vi "VI Stoermeldung Konfig.vi"() -> ()   [LabVIEW 2020, in "Stoerungen.lvlib"]
uses:
  Stoerungen/Stoerungen.lvlib
  Stoerungen/Stoermeldung Konfig Anzeige.ctl
  Stoerungen/Stoermeldung Konfig.ctl
  Visualisierungs Elemente/Zahlen-Ausgabefeld.ctl
  Visualisierungs Elemente/Zahlen-Eingabefeld.ctl
  Visualisierungs Elemente/String - Ausgabefeld.ctl
  Visualisierungs Elemente/Button.ctl
  Sprachverwaltung/FGV Aktion Tabelle zerlegen.ctl
  Passwortverwaltung/FGV Passwort Aktion.ctl
  Stoerungen/FGV Stoerungsdatei Aktionen.ctl
  Stoerungen/FGV Stoerung aufnehmen Aktion.ctl
  Passwortverwaltung/Passwort.lvlib
  Allgemein/allgemeine Sub-VIs.lvlib
  Sprachverwaltung/Sprachverwaltung.lvlib
panel:
  in  "Speichern":T1
  in  "Konfig":T2 {"Ansprech" format="%#_5g"; "Nummer" format="%#_5g"}
  # "Störmeldungs-Konfiguration"
  # "Störungs-\nNummer"
  # "Ansprech-\nverzögerung"
  # "Quittieren"
  # "Abschalten"
  # "Meldung"
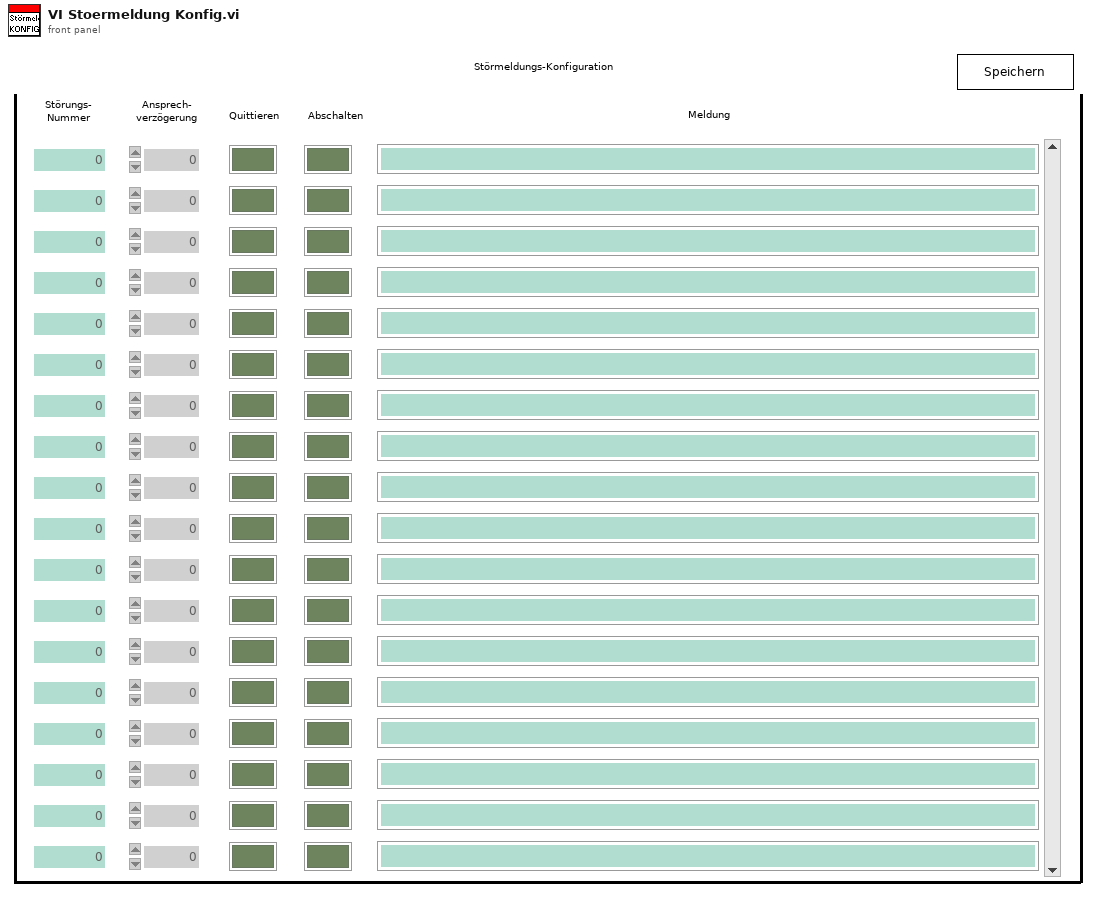
[diagram p1: front panel]
types:
  T1 = typedef "Button.ctl" = bool
  T2 = typedef "Stoerungen.lvlib/Stoermeldung Konfig Anzeige.ctl" = T3[]
  T3 = typedef "Stoerungen.lvlib/Stoermeldung Konfig.ctl" = cluster{"Quitt":bool, "Stopp":bool, "Nummer":T4, "Ansprech":T5, "Meldung":T6}
  T4 = typedef "Zahlen-Ausgabefeld.ctl" = sgl
  T5 = typedef "Zahlen-Eingabefeld.ctl" = sgl
  T6 = typedef "String - Ausgabefeld.ctl" = string
  T7 = typedef "Sprachverwaltung.lvlib/FGV Aktion Tabelle zerlegen.ctl" = enum16{"laden", "vereinzeln", "speichern"}
  T8 = typedef "Passwort.lvlib/FGV Passwort Aktion.ctl" = enum16{"prüfen", "setzen", "Initialisieren", "PW speichern", "lesen", "PW Änderung"}
  T9 = enum16{"open", "replace", "create", "open or create", "replace or create", "replace or create with confirmation"}
  T10 = typedef "Stoerungen.lvlib/FGV Stoerungsdatei Aktionen.ctl" = enum16{"lesen", "laden", "Neue Werte"}
  T11 = typedef "Stoerungen.lvlib/FGV Stoerung aufnehmen Aktion.ctl" = enum16{"Initialisieren", "Schreiben", "Lesen", "Quittieren", "quit. löschen"}
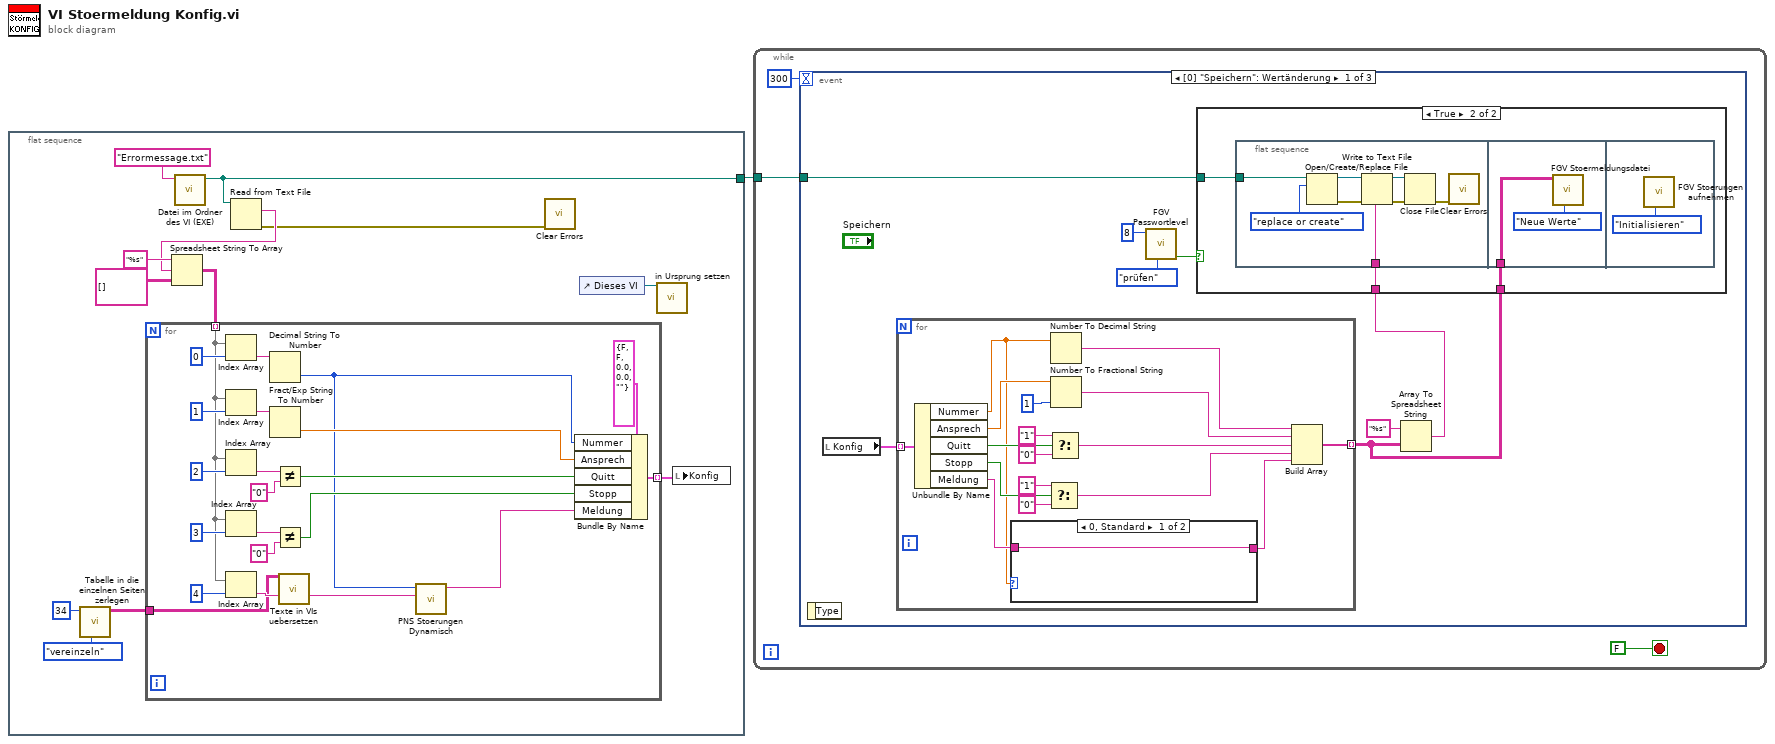
[diagram p0: block diagram]
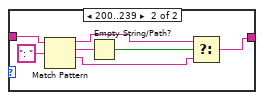
[diagram p3: hidden frame]
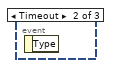
[diagram p4: hidden frame]
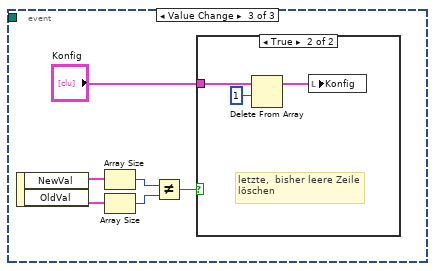
[diagram p5: hidden frame]
diagram:
  n1 = flat-sequence {
    tunnel: [w9] -> w1
    frame #0 {
      n2 = call "Tabelle in die einzelnen Seiten zerlegen.vi"("Aktion"=FGV_Aktion_Tabelle_zerlegen."vereinzeln", "Index (Seite)"=34) -> ("Sprachliste"=w3:string[][])  [unwired: 7 in, 2 out]
      n3 = call "Datei im Ordner des VI (EXE).vi"("Dateiname"="Errormessage.txt") -> ("Dateipfad im Ordner des Haupt-VIs"=w9:path)  [unwired: 8 in, 2 out]
      n4 = Read from Text File(file (use dialog)=w9) -> (text=w7:string, error out=w6:errorcluster)  [unwired: 1 in, 4 out]
      n5 = Spreadsheet String To Array(format string="%s" ("Format-String"), spreadsheet string=w7, array type (2D Dbl)=string[][] []) -> (array=w10:string[][])  [unwired: 1 out]
      n6 = for {
        tunnel: w10 -> [w27] mode=indexing
        tunnel: [w19] -> w8 mode=indexing
        tunnel: w3 -> [w17]
        n7 = Index Array(array=w27, index=0 ("Index")) -> (element=w24:string)
        n8 = Index Array(array=w27, index=1 ("Index")) -> (element=w31:string)
        n9 = Index Array(array=w27, index=2 ("Index")) -> (element=w34:string)
        n10 = Index Array(array=w27, index=3 ("Index")) -> (element=w30:string)
        n11 = Index Array(array=w27, index=4 ("Index")) -> (element=w18:string)
        n12 = Decimal String To Number(string=w24) -> (number=w15:i32)  [unwired: 3 out]
        n13 = Fract/Exp String To Number(string=w31) -> (number=w22:dbl)  [unwired: 4 out]
        n14 = Not Equal?(x=w34, y="0") -> (x != y?=w21:bool)
        n15 = Not Equal?(x=w30, y="0") -> (x != y?=w20:bool)
        n16 = call "Texte in VIs uebersetzen.vi"("Sprachliste"=w17, "String zum Übersetzen"=w18) -> ("String zum Übersetzen"=w16:string)  [unwired: 9 in, 4 out]
        n17 = call "PNS Stoerungen Dynamisch.vi"("Störmeldetexte"=w16, "Nummer"=w15) -> ("String"=w14:string)  [unwired: 9 in]
        n18 = Bundle By Name(cluster=T3 {"Quitt"=FALSE, "Stopp"=FALSE, "Nummer"=0.0, "Ansprech"=0.0, "Meldung"=""} ("Störmeldung Konfig"), "Nummer"=w15, "Ansprech"=w22, "Quitt"=w21, "Stopp"=w20, "Meldung"=w14) -> (w19:T3)
      }
      n19 = call <vilib>:"Clear Errors.vi"("error in (no error)"=w6) -> ()  [unwired: 5 in, 2 out]
      n20 = control-ref of="Dieses VI"() -> (w5:refnum<vi>)
      n21 = call "in Ursprung setzen.vi"("VI Referenz"=w5) -> ()  [unwired: 10 in, 1 out]
      n22 = local write "Konfig"(w8) -> ()
    }
  }
  n23 = while {
    tunnel: w1 -> [w38]
    stop <- FALSE stop-if-true
    n24 = event shown="[0] \"Speichern\": Wertänderung" {
      selector: _ -> [_ _ _]
      dyn-events: _ -> [_ _ _]
      timeout: 300 -> [_ _ _]
      tunnel: w38 -> [w46 _ _]
      event Value Change {
        n25 = event-data() -> ()  [unwired: 2 out]
        n26 = local read "Konfig"() -> (w43:T2)
        n27 = for {
          tunnel: [w77] -> w39 mode=indexing
          tunnel: w43 -> [w76] mode=indexing
          n28 = Unbundle By Name(w76) -> ("Nummer"=w62:T4, "Ansprech"=w73:T5, "Quitt"=w75:bool, "Stopp"=w74:bool, "Meldung"=w63:T6)
          n29 = case shown="0, Standard" w62 {
            tunnel: w63 -> [w78 w84]
            tunnel: [w78 w80] -> w61
            frame 0, Default {
            }
            frame 200..239 {
              n30 = Match Pattern(string=w84, regular expression=": " ("Regulärer Ausdruck")) -> (before substring=w82:T6, match substring=w81:T6, after substring=w79:T6)  [unwired: 1 in, 1 out]
              n31 = Empty String/Path?(string/path=w81) -> (empty?=w83:bool)
              n32 = Select(t=w82, s=w83, f=w79) -> (s? t:f=w80:T6)
            }
          }
          n33 = Select(t="1", s=w74, f="0") -> (s? t:f=w64:string)
          n34 = Select(t="1", s=w75, f="0") -> (s? t:f=w65:string)
          n35 = Number To Decimal String(number=w62) -> (decimal integer string=w72:string)  [unwired: 1 out]
          n36 = Number To Fractional String(number=w73, precision (6)=i16 1 ("Genauigkeit (6)")) -> (F-format string=w67:string)  [unwired: 2 out]
          n37 = Build Array(w72, w67, w65, w64, w61) -> (w77:T6[])
        }
        n38 = call "FGV Passwortlevel.vi"("FGV Passwort Aktion"=FGV_Passwort_Aktion."prüfen", "geforderter Level"=i16 8) -> ("Freigabe"=w41:bool)  [unwired: 2 in, 7 out]
        n39 = Array To Spreadsheet String(array=w39, 3:"%s" ("Format-String")) -> (spreadsheet string=w44:string)  [unwired: 1 out]
        n40 = case shown="True" w41 {
          tunnel: w46 -> [_ w49]
          tunnel: w44 -> [_ w48]
          tunnel: w39 -> [_ w47]
          frame False {
          }
          frame True {
            n41 = flat-sequence {
              tunnel: w49 -> [w57]
              tunnel: w48 -> [w56]
              tunnel: w47 -> [w58]
              frame #0 {
                n42 = Open/Create/Replace File(file path (use dialog)=w57, operation (0:open)=T9."replace or create" ("Operation (0:Öffnen)")) -> (refnum out=w53:refnum<file>, error out=w52:errorcluster)  [unwired: 1 in, 4 out]
                n43 = Write to Text File(file (use dialog)=w53, text=w56, error in=w52) -> (refnum out=w55:refnum<file>, error out=w51:errorcluster)  [unwired: 2 out]
                n44 = Close File(refnum=w55, error in=w51) -> (error out=w50:errorcluster)  [unwired: 1 out]
                n45 = call <vilib>:"Clear Errors.vi"("error in (no error)"=w50) -> ()  [unwired: 5 in, 2 out]
              }
              frame #1 {
                n46 = call "FGV Stoermeldungsdatei.vi"("Aktionen"=FGV_Stoerungsdatei_Aktionen."Neue Werte", "Neue Tabelle"=w58) -> ()  [unwired: 1 in, 9 out]
              }
              frame #2 {
                n47 = call "FGV Stoerungen aufnehmen.vi"("FGV Störung aufnehmen Aktion"=FGV_Stoerung_aufnehmen_Aktion."Initialisieren") -> ()  [unwired: 7 in, 4 out]
              }
            }
          }
        }
      }
      event Timeout {
        n48 = event-data() -> ()  [unwired: 2 out]
      }
      event Value Change {
        n49 = event-data() -> ("NewVal"=w91:T2, "OldVal"=w90:T2)  [unwired: 1 out]
        n50 = Array Size(array=w91) -> (size(s)=w89:i32)
        n51 = Array Size(array=w90) -> (size(s)=w88:i32)
        n52 = Not Equal?(x=w89, y=w88) -> (x != y?=w86:bool)
        n53 = case shown="True" w86 {
          tunnel: "Konfig" -> [_ w94]
          frame False {
          }
          frame True {
            # "letzte,  bisher leere Zeile\nlöschen"
            n54 = Delete From Array(array=w94, length=1 ("Länge")) -> (array with subset deleted=w92:T2)  [unwired: 1 in, 1 out]
            n55 = local write "Konfig"(w92) -> ()
          }
        }
      }
    }
  }
